vi "Enk_Skalowanie drogi GUI.vi"(8 "error in (no error)":errorcluster, 10 "Droga In":dbl) -> (0 "error out":errorcluster, 2 "Skala":dbl)   [LabVIEW 2013]
doc: "Wprowadza wartoœæ skali dla enkodera"
panel:
  out "Wskazanie":dbl
  in  "Przebyta droga":dbl
  in  "Cancel":bool
  in  "OK":bool
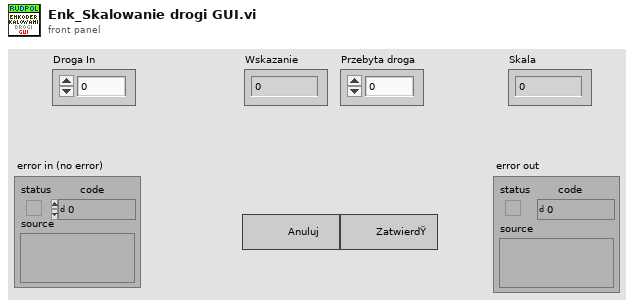
[diagram p1: front panel]
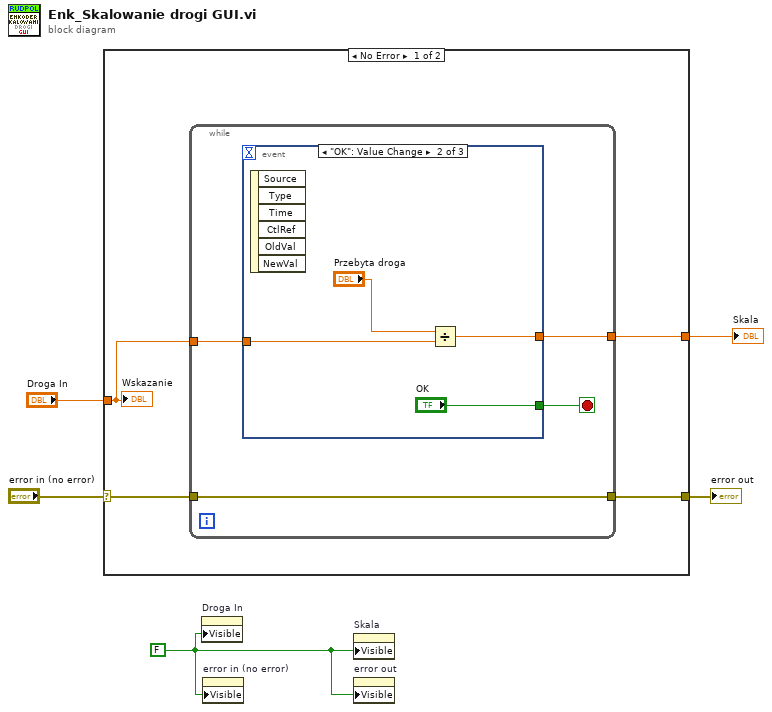
[diagram p0: block diagram]
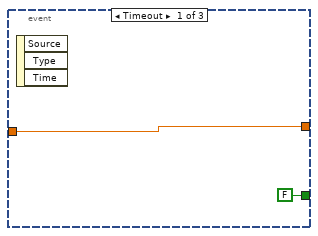
[diagram p2: hidden frame]
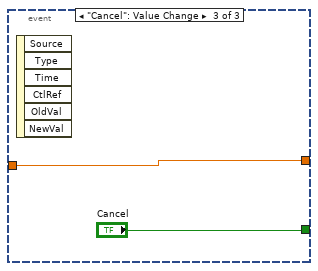
[diagram p3: hidden frame]
diagram:
  w1 = FALSE ("Visible")
  n1 = case shown="No Error" "error in (no error)" {
    selector: "error in (no error)" -> [w8 w23]
    tunnel: [w9 w23] -> w4
    tunnel: "Droga In" -> [w7 w22]
    tunnel: [w6 w22] -> w2
    frame No Error {
      n2 = while {
        tunnel: [w13] -> w9
        tunnel: w8 -> [w13]
        tunnel: w7 -> [w12]
        tunnel: [w10] -> w6
        stop <- w11 stop-if-true
        n3 = event shown="[1] \"OK\": Value Change" {
          selector: _ -> [_ _ _]
          dyn-events: _ -> [_ _ _]
          timeout: _ -> [_ _ _]
          tunnel: w12 -> [w15 w17 w21]
          tunnel: [FALSE ("OK") "OK" "Cancel"] -> w11
          tunnel: [w15 w16 w21] -> w10
          event Timeout {
            n4 = event-data() -> ()  [unwired: 1 in, 3 out]
          }
          event "OK": Value Change {
            n5 = event-data() -> ()  [unwired: 1 in, 6 out]
            n6 = Divide(x="Przebyta droga", y=w17) -> (x/y=w16:dbl)
          }
          event "Cancel": Value Change {
            n7 = event-data() -> ()  [unwired: 1 in, 6 out]
          }
        }
      }
      "Wskazanie" <- w7
    }
    frame Error {
    }
  }
  "error out" <- w4
  "Skala" <- w2
  n8 = property on="Droga In" class="DigNum (strict)"("Visible"=w1) -> ()  [unwired: 2 in, 2 out]
  n9 = property on="error in (no error)" class="Clust (strict)"("Visible"=w1) -> ()  [unwired: 2 in, 2 out]
  n10 = property on="Skala" class="DigNum (strict)"("Visible"=w1) -> ()  [unwired: 2 in, 2 out]
  n11 = property on="error out" class="Clust (strict)"("Visible"=w1) -> ()  [unwired: 2 in, 2 out]
